vi "Set sub-Item by names.vi"(8 "error in (no error)":errorcluster, 9 "Value":refnum<class "JSON Value.lvclass">, 10 "Name Array":string[](array[string]), 11 "JSON Value In":refnum<class "JSON Value.lvclass">) -> (0 "error out":errorcluster, 1 "replaced":bool, 3 "JSON Value Out":refnum<class "JSON Value.lvclass">)   [LabVIEW 2020, in "Library Commun.lvlib" / "JSON Value.lvclass"]
doc: "Sets a JSON object in a JSON collection by it's path (an array of strings).\n\nCopyright 2012 James David Powell, Shaun Rumbell and Ton Plomp\nMore information on http://lavag.org/topic/16217-cr-json-labview"
uses:
  JSON Value.lvclass
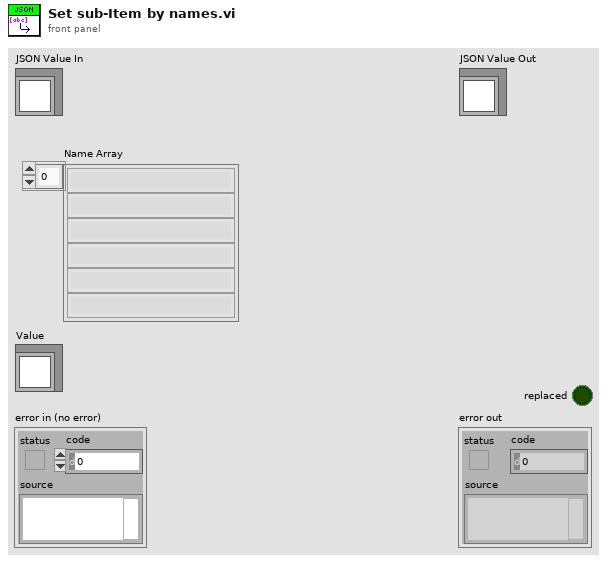
[diagram p1: front panel]
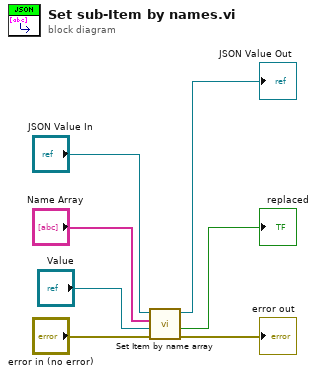
[diagram p0: block diagram]
diagram:
  n1 = call "Set Item by name array.vi"("error in (no error)"="error in (no error)", "Value"="Value", "Name Array"="Name Array", "JSON Value In"="JSON Value In") -> ("error out"=→"error out":errorcluster, "replaced"=→"replaced":bool, "JSON Value Out"=→"JSON Value Out":refnum<class "JSON Value.lvclass">)  [unwired: 5 in]
